vi "strings to line.vi"(11 "strings":string[](array[string])) -> (3 "line":T1)   [LabVIEW 2013, in "TEC editor node.lvclass"]
uses:
  TEC editor node.lvclass
  table line.ctl
  <vilib>/NI/Tag Bus Module Framework/channel/TBM channel.lvclass
  <vilib>/NI/Tag Bus/tag/Data Type.ctl
  permissions.ctl
  <vilib>/NI/Tag Bus/tag/tag descriptor.lvclass/tag descriptor.ctl
  <vilib>/NI/Tag Bus Module Framework/channel/TBM channel.lvclass/TBM channel.ctl
  <vilib>/NI/Tag Bus/tag/write tag name.vi
  <vilib>/NI/Tag Bus Module Framework/channel/Write channel classification.vi
  <vilib>/NI/Tag Bus/tag/write data type.vi
  <vilib>/NI/Tag Bus/tag/tag descriptor.lvclass
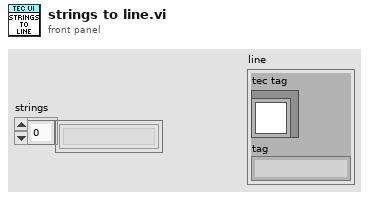
[diagram p1: front panel]
types:
  T1 = typedef "TEC editor node.lvclass/table line.ctl" = cluster{"tec tag":refnum<class "TBM channel.lvclass">, "tag":string}
  T2 = typedef "TEC editor node.lvclass/permissions.ctl" = enum16{"Read from Ext Engine", "Write to Ext Engine"}
  T3 = typedef "tag bus.lvlib/tag descriptor.lvclass/Data Type.ctl" = enum16{"Double", "Single", "I64", "I32", "I16", "I8", "U64", "U32", "U16", "U8", "Boolean", "String", "Array of Double", "Array of Single", "Array of I64", "Array of I32", "Array of I16", "Array of I8", "Array of U64", "Array of U32", "Array of U16", "Array of U8", "Array of Boolean", "Array of String"}
  T4 = typedef "TBM channel.lvclass/channel classification.ctl" = enum16{"input data", "output data", "processing parameter", "processing result"}
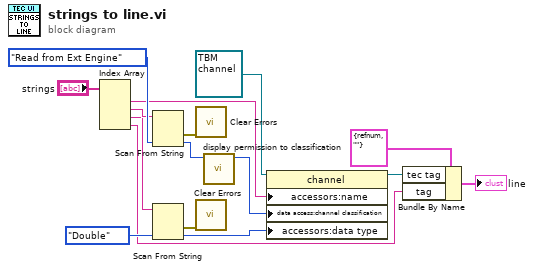
[diagram p0: block diagram]
diagram:
  n1 = Index Array(array="strings") -> (element #1=w1:string, element #2=w9:string, element #3=w7:string, element #4=w6:string)  [unwired: 4 in]
  n2 = Scan From String(input string=w9, default 1=permissions."Read from Ext Engine" ("direction")) -> (error out=w11:errorcluster, output 1=w8:T2)  [unwired: 3 in, 2 out]
  n3 = Scan From String(input string=w7, default 1=Data_Type."Double" ("data type")) -> (error out=w13:errorcluster, output 1=w3:T3)  [unwired: 3 in, 2 out]
  n4 = call <vilib>:"Clear Errors.vi"("error in (no error)"=w11) -> ()  [unwired: 6 in, 1 out]
  n5 = call <vilib>:"Clear Errors.vi"("error in (no error)"=w13) -> ()  [unwired: 6 in, 1 out]
  n6 = call "display permission to classification.vi"("display permissions"=w8) -> ("channel classification"=w2:T4)  [unwired: 10 in]
  n7 = property class="channel"(reference=refnum<class "TBM channel.lvclass"> refnum ("channel"), "accessors:name"=w1, "data access:channel classification"=w2, "accessors:data type"=w3) -> (reference out=w4:refnum<class "TBM channel.lvclass">)  [unwired: 1 in, 1 out]
  n8 = Bundle By Name(cluster=T1 {"tec tag"=refnum, "tag"=""} ("line"), "tec tag"=w4, "tag"=w6) -> (→"line":T1)
